vi "rescale_PI_gains.vi"(9 "Dinv-k":dbl, 11 "z-axis-params-in":T1={"z_u_max"=5.0, "setpoint_scan"=0.0, "Ki_scan"=0.001, "uz_safe"=0.0, "Kiz_down"=0.001, "setpoint_up"=0.0, "do_Dz"=FALSE, "PID_while_xy_move"=FALSE, "TF_params"={"TF_order"=0, "Num"=[0.0, 0.0, 0.0, 0.0, 0.0, 0.0, 0.0, 0.0, 0.0], "Den"=[0.0, 0.0, 0.0, 0.0, 0.0, 0.0, 0.0, 0.0, 0.0]}} {"uz_safe" format="%#_13g"}) -> (0 "Kiscan-effective":dbl, 1 "Kidown-effective":dbl, 3 "z-axis-params-out":T1={"z_u_max"=5.0, "setpoint_scan"=0.0, "Ki_scan"=0.001, "uz_safe"=0.0, "Kiz_down"=0.001, "setpoint_up"=0.0, "do_Dz"=FALSE, "PID_while_xy_move"=FALSE, "TF_params"={"TF_order"=0, "Num"=[0.0, 0.0, 0.0, 0.0, 0.0, 0.0, 0.0, 0.0, 0.0], "Den"=[0.0, 0.0, 0.0, 0.0, 0.0, 0.0, 0.0, 0.0, 0.0]}} {"uz_safe" format="%#_13g"})   [LabVIEW 2019]
uses:
  controls/z-axis-params_v4_prescan.ctl
  controls/TF-params.ctl
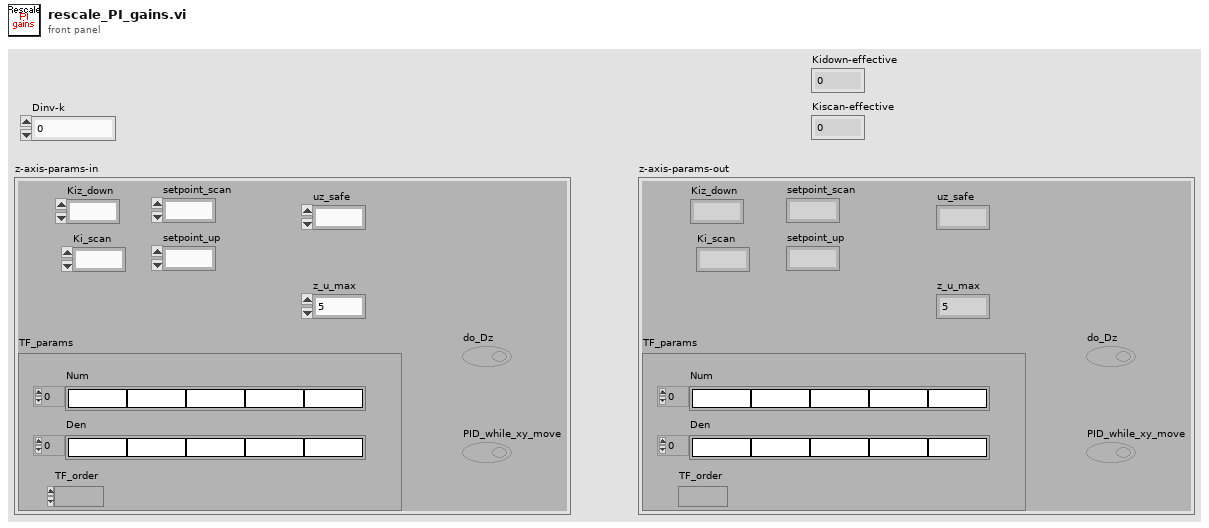
[diagram p1: front panel]
types:
  T1 = typedef "z-axis-params_v4_prescan.ctl" = cluster{"z_u_max":sgl, "setpoint_scan":fxp<+/-,32,16>, "Ki_scan":sgl, "uz_safe":fxp<+/-,16,5>, "Kiz_down":sgl, "setpoint_up":fxp<+/-,32,16>, "do_Dz":bool, "PID_while_xy_move":bool, "TF_params":T2}
  T2 = typedef "TF-params.ctl" = cluster{"TF_order":i16, "Num":sgl[], "Den":sgl[]}
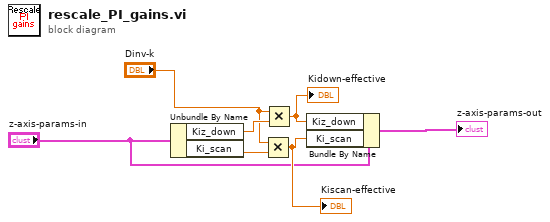
[diagram p0: block diagram]
diagram:
  n1 = Unbundle By Name("z-axis-params-in") -> ("Kiz_down"=w6:sgl, "Ki_scan"=w7:sgl)
  n2 = Multiply(x="Dinv-k", y=w7) -> (x*y=w4:dbl)
  "Kiscan-effective" <- w4
  n3 = Multiply(x="Dinv-k", y=w6) -> (x*y=w3:dbl)
  "Kidown-effective" <- w3
  n4 = Bundle By Name(cluster="z-axis-params-in", "Kiz_down"=w3, "Ki_scan"=w4) -> (→"z-axis-params-out":T1)
